vi "Configure Composite Limit Test.vi"(0 "VISA resource name":refnum<visa-resource-name>, 1 "Enable Composite Limit Test (F: Disable)":bool, 2 "CLimit Fail Result Pattern (16383)":i32=16383, 3 "CLimit  Result Update Mode (0: Immediate)":i32(ring) items=["Immediate", "END"], 5 "Channel (0: Channel 1)":i32(ring) items=["Channel 1", "Channel 2"], 9 "CLimit Operation Mode (0: Grading)":i32(ring) items=["Grading", "Sort"], 11 "error in (no error)":errorcluster, 13 "CLimit Pass Result Pattern (16383)":i32=16383, 14 "Limit Test Feed Mode (0: Voltage)":i32(ring) items=["Voltage", "Current", "Resistance", "Math"]) -> (4 "VISA resource name out":refnum<visa-resource-name>, 15 "error out":errorcluster)   [LabVIEW 2020, in "Agilent B2900 Series.lvlib"]
doc: "Change the settings for composite limit test.\nIf you want to use the GPIO port for sending a pass/fail bit pattern, use Configure CLT GPIO Pins.vi.\nIf you want to use the null offset for cancelling the offset value from the\nmeasurement data automatically, use Configure Limit Test Null Offset.vi.\n\n<B>Note:</B>\nCommands in default part of the case structure are not applicable for Agilent models B2961A, B2962A, B2961B and B2962B."
uses:
  Agilent B2900 Series.lvlib
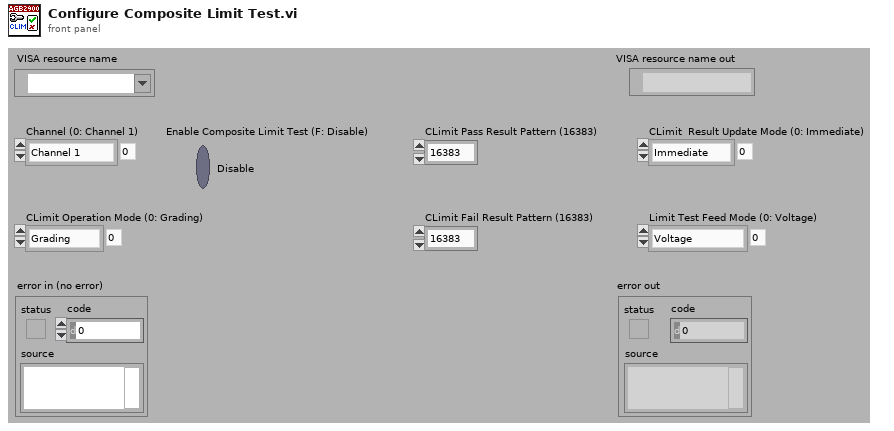
[diagram p1: front panel]
types:
  T1 = typedef "Agilent B2900 Series.lvlib/Extended User Data.ctl" = cluster{"B2900 Series Mode":u16}
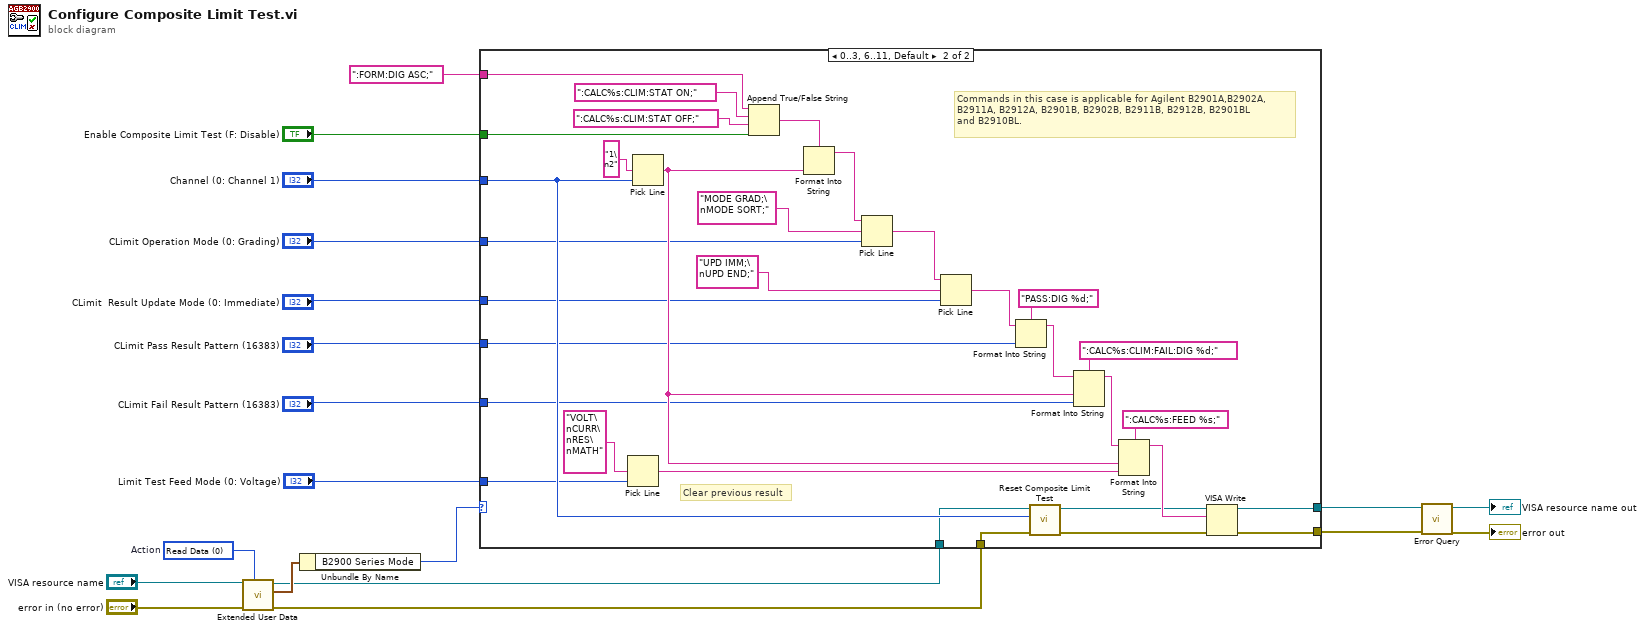
[diagram p0: block diagram]
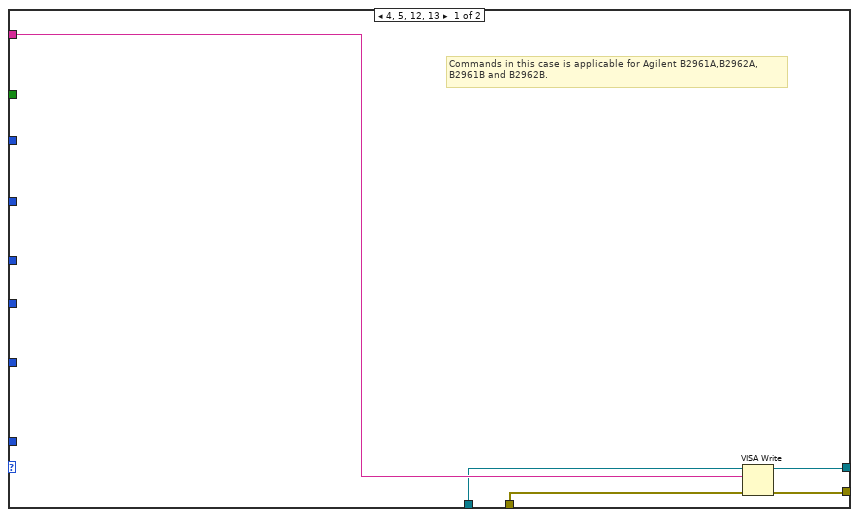
[diagram p2: hidden frame]
diagram:
  w16 = 0 items=["Read Data", "Write Data", "Clear Data", "Clear ALL Data"]  # Action
  n1 = call "Extended User Data.vi"("Action (1: Write Data)"=w16, "Error In (no error)"="error in (no error)", "VISA resource name in"="VISA resource name") -> ("Error Out"=w4:errorcluster, "User Data Out"=w15:T1, "VISA resource name out"=w5:refnum<visa-resource-name>)  [unwired: 6 in]
  n2 = Unbundle By Name(w15) -> ("B2900 Series Mode"=w14:u16)
  n3 = case shown="0..3, 6..11, Default" w14 {
    tunnel: "Enable Composite Limit Test (F: Disable)" -> [_ w39]
    tunnel: "Channel (0: Channel 1)" -> [_ w38]
    tunnel: "CLimit Operation Mode (0: Grading)" -> [_ w37]
    tunnel: "CLimit  Result Update Mode (0: Immediate)" -> [_ w36]
    tunnel: "CLimit Pass Result Pattern (16383)" -> [_ w35]
    tunnel: "CLimit Fail Result Pattern (16383)" -> [_ w34]
    tunnel: "Limit Test Feed Mode (0: Voltage)" -> [_ w33]
    tunnel: ":FORM:DIG ASC;" -> [w24 w32]
    tunnel: w5 -> [w22 w31]
    tunnel: w4 -> [w23 w30]
    tunnel: [w21 w26] -> w3
    tunnel: [w20 w25] -> w2
    frame 4, 5, 12, 13 {
      # "Commands in this case is applicable for Agilent B2961A,B2962A,\nB2961B and B2962B."
      n4 = VISA Write(VISA resource name=w22, write buffer=w24, error in (no error)=w23) -> (VISA resource name out=w21:refnum<visa-resource-name>, error out=w20:errorcluster)  [unwired: 1 out]
    }
    frame 0..3, 6..11, Default {
      # "Commands in this case is applicable for Agilent B2901A,B2902A,\nB2911A, B2912A, B2901B, B2902B, B2911B, B2912B, B2901BL \nand B2910BL."
      # "Clear previous result"
      n5 = Pick Line(multi-line string="VOLT\nCURR\nRES\nMATH", line index=w33) -> (output string=w54:string)  [unwired: 1 in]
      n6 = Pick Line(multi-line string="1\n2" ("string (\"\")"), line index=w38) -> (output string=w56:string)  [unwired: 1 in]
      n7 = Append True/False String(1:w39, 2:":CALC%s:CLIM:STAT OFF;", 3:":CALC%s:CLIM:STAT ON;", 4:w32) -> (0:w48:string)
      n8 = Format Into String(format string=w48, w56) -> (resulting string=w51:string)  [unwired: 2 in, 1 out]
      n9 = Pick Line(string ("")=w51, multi-line string="MODE GRAD;\nMODE SORT;", line index=w37) -> (output string=w50:string)
      n10 = Pick Line(string ("")=w50, multi-line string="UPD IMM;\nUPD END;", line index=w36) -> (output string=w44:string)
      n11 = Format Into String(format string="PASS:DIG %d;", initial string=w44, w35) -> (resulting string=w49:string)  [unwired: 1 in, 1 out]
      n12 = call "Reset Composite Limit Test.vi"("error in (no error)"=w30, "Channel (0: Channel 1)"=w38, "VISA resource name"=w31) -> ("error out"=w27:errorcluster, "VISA resource name out"=w28:refnum<visa-resource-name>)  [unwired: 7 in]
      n13 = Format Into String(format string=":CALC%s:CLIM:FAIL:DIG %d;", initial string=w49, w56, w34) -> (resulting string=w55:string)  [unwired: 1 in, 1 out]
      n14 = Format Into String(format string=":CALC%s:FEED %s;", initial string=w55, w56, w54) -> (resulting string=w29:string)  [unwired: 1 in, 1 out]
      n15 = VISA Write(VISA resource name=w28, write buffer=w29, error in (no error)=w27) -> (VISA resource name out=w26:refnum<visa-resource-name>, error out=w25:errorcluster)  [unwired: 1 out]
    }
  }
  n16 = call "Error Query.vi"("error in (no error)"=w2, "VISA resource name"=w3) -> ("error out"=→"error out":errorcluster, "VISA resource name out"=→"VISA resource name out":refnum<visa-resource-name>)  [unwired: 6 in, 2 out]
